vi "Gateway_SetupSSH.vi"(0 "GatewayClass in":refnum<class "GatewayClass.lvclass">, 1 "ssh hostname":string, 2 "ssh host port":i32=22, 3 "username":string, 4 "password":string, 5 "error in (no error)":errorcluster) -> (14 "GatewayClass out":refnum<class "GatewayClass.lvclass">, 19 "error out":errorcluster)   [LabVIEW 2018, in "GatewayClass.lvclass"]
uses:
  GatewayClass.lvclass
  GatewayClass.lvclass/GatewayClass.ctl
  DataPacker/Utilities/SSH_TUNNEL.lvclass/SSH_TUNNEL.ctl
  DataPacker/Utilities/SSH_TUNNEL.lvclass
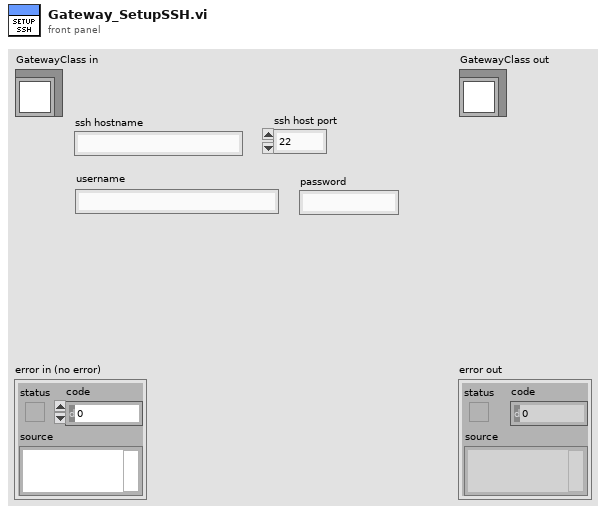
[diagram p1: front panel]
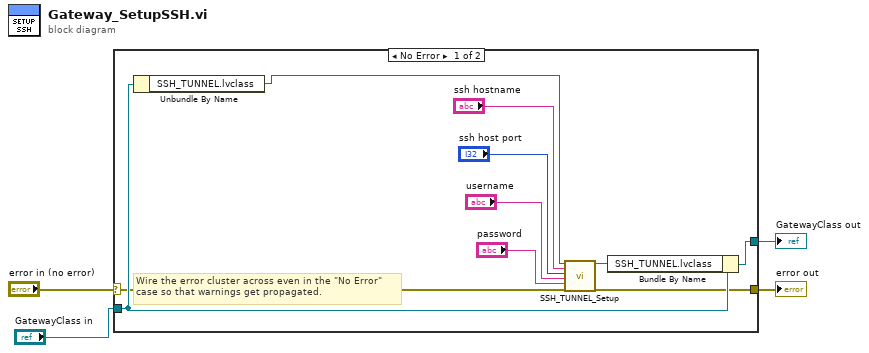
[diagram p0: block diagram]
diagram:
  n1 = case shown="No Error" "error in (no error)" {
    selector: "error in (no error)" -> [w7 w16]
    tunnel: [w8 w16] -> w3
    tunnel: [w10 w15] -> w1
    tunnel: "GatewayClass in" -> [w11 w15]
    frame No Error {
      # "Wire the error cluster across even in the \"No Error\"\ncase so that warnings get propagated."
      n2 = Unbundle By Name(w11) -> ("SSH_TUNNEL.lvclass"=w12:refnum<class "SSH_TUNNEL.lvclass">)
      n3 = call "SSH_TUNNEL_Setup.vi"("SSH_TUNNEL in"=w12, "ssh hostname"="ssh hostname", "ssh host port"="ssh host port", "username"="username", "password"="password", "error in (no error)"=w7) -> ("SSH_TUNNEL out"=w9:refnum<class "SSH_TUNNEL.lvclass">, "error out"=w8:errorcluster)  [unwired: 12 in]
      n4 = Bundle By Name(cluster=w11, "SSH_TUNNEL.lvclass"=w9) -> (w10:refnum<class "GatewayClass.lvclass">)
    }
    frame Error {
    }
  }
  "error out" <- w3
  "GatewayClass out" <- w1
